vi "DraggingDresser.vi"() -> ()   [LabVIEW 2015]
panel:
  out "Force":dbl[](array[numeric])=[1.0, 0.9829941021665359, 0.9668465198454019, 0.9515060280912325, 0.9369256727572303, 0.9230623464972036, 0.9098764147997167, 0.8973313853270691, 0.8853936148477479, 0.8740320488976421, 0.8632179900134445, 0.8529248909760372, 0.8431281700022195, 0.8338050452460644, 0.8249343863296593, 0.8164965809277261, 0.8084734146904488, 0.8008479630110114, 0.7936044933348412, 0.7867283768713176, 0.7802060087098789, 0.7740247354644318, 0.768172789675662, 0.7626392302926074, 0.7574138886347647, 0.7524873193057124, 0.7478507555902304, 0.743496068920369, 0.7394157320429343, 0.7356027855622788, 0.7320508075688773, 0.7287538860965921, 0.7257065941803166, 0.7229039673113511, 0.7203414831107795, 0.7180150430616907, 0.7159209561595877, 0.714055924357065, 0.7124170296940266, 0.7110017230185812, 0.7098078142164795, 0.7088334638787107, 0.7080771763478116, 0.7075377940936781, 0.7072144933793596, 0.7071067811865476, 0.7072144933793596, 0.7075377940936781, 0.7080771763478118, 0.7088334638787107, 0.7098078142164794, 0.7110017230185813, 0.7124170296940266, 0.7140559243570649, 0.7159209561595877, 0.7180150430616907, 0.7203414831107795, 0.7229039673113511, 0.7257065941803166, 0.728753886096592, 0.7320508075688772, 0.7356027855622788, 0.7394157320429343, 0.743496068920369, 0.7478507555902304, 0.7524873193057124, 0.7574138886347643, 0.7626392302926074, 0.768172789675662, 0.774024735464432, 0.7802060087098789, 0.7867283768713176, 0.7936044933348411, 0.8008479630110114, 0.8084734146904488, 0.8164965809277261, 0.8249343863296593, 0.8338050452460642, 0.8431281700022196, 0.8529248909760372, 0.8632179900134445, 0.8740320488976421, 0.8853936148477479, 0.8973313853270691, 0.9098764147997167, 0.9230623464972035, 0.9369256727572305, 0.9515060280912323, 0.9668465198454019, 0.9829941021665357, 1.0]
  out "Angle for Minimum Force":i32=45 format="%.1f"
  in  "Coefficient of Kinetic Friction":dbl=1.0 format="%.1f"
  out "Waveform Graph":dbl[](graph)=[1.0, 0.9829941021665359, 0.9668465198454019, 0.9515060280912325, 0.9369256727572303, 0.9230623464972036, 0.9098764147997167, 0.8973313853270691, 0.8853936148477479, 0.8740320488976421, 0.8632179900134445, 0.8529248909760372, 0.8431281700022195, 0.8338050452460644, 0.8249343863296593, 0.8164965809277261, 0.8084734146904488, 0.8008479630110114, 0.7936044933348412, 0.7867283768713176, 0.7802060087098789, 0.7740247354644318, 0.768172789675662, 0.7626392302926074, 0.7574138886347647, 0.7524873193057124, 0.7478507555902304, 0.743496068920369, 0.7394157320429343, 0.7356027855622788, 0.7320508075688773, 0.7287538860965921, 0.7257065941803166, 0.7229039673113511, 0.7203414831107795, 0.7180150430616907, 0.7159209561595877, 0.714055924357065, 0.7124170296940266, 0.7110017230185812, 0.7098078142164795, 0.7088334638787107, 0.7080771763478116, 0.7075377940936781, 0.7072144933793596, 0.7071067811865476, 0.7072144933793596, 0.7075377940936781, 0.7080771763478118, 0.7088334638787107, 0.7098078142164794, 0.7110017230185813, 0.7124170296940266, 0.7140559243570649, 0.7159209561595877, 0.7180150430616907, 0.7203414831107795, 0.7229039673113511, 0.7257065941803166, 0.728753886096592, 0.7320508075688772, 0.7356027855622788, 0.7394157320429343, 0.743496068920369, 0.7478507555902304, 0.7524873193057124, 0.7574138886347643, 0.7626392302926074, 0.768172789675662, 0.774024735464432, 0.7802060087098789, 0.7867283768713176, 0.7936044933348411, 0.8008479630110114, 0.8084734146904488, 0.8164965809277261, 0.8249343863296593, 0.8338050452460642, 0.8431281700022196, 0.8529248909760372, 0.8632179900134445, 0.8740320488976421, 0.8853936148477479, 0.8973313853270691, 0.9098764147997167, 0.9230623464972035, 0.9369256727572305, 0.9515060280912323, 0.9668465198454019, 0.9829941021665357, 1.0]
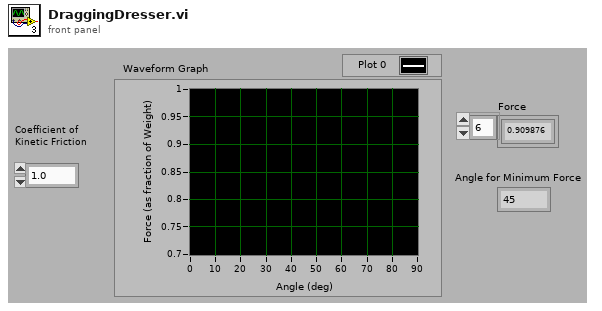
[diagram p1: front panel]
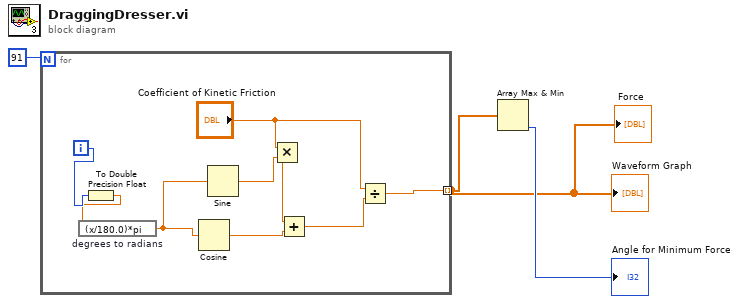
[diagram p0: block diagram]
diagram:
  n1 = for {
    N: 91 -> [_]
    tunnel: [w7] -> w1 mode=indexing
    i -> [w5]
    n2 = To Double Precision Float(number=w5) -> (double precision float=w4:dbl)
    n3 = expression code="(x/180.0)*pi" "degrees to radians"(w4) -> (w6:dbl)
    n4 = Cosine(x=w6) -> (cos(x)=w12:dbl)
    n5 = Sine(x=w6) -> (sin(x)=w11:dbl)
    n6 = Multiply(x="Coefficient of Kinetic Friction", y=w11) -> (x*y=w10:dbl)
    n7 = Add(x=w10, y=w12) -> (x+y=w9:dbl)
    n8 = Divide(x="Coefficient of Kinetic Friction", y=w9) -> (x/y=w7:dbl)
  }
  "Waveform Graph" <- w1
  "Force" <- w1
  n9 = Array Max & Min(array=w1) -> (min index (indices)=→"Angle for Minimum Force":i32)  [unwired: 3 out]
